vi "Write States.vi"(8 "error in (no error)":errorcluster, 10 "States":T1, 11 "MarkerTactic in":refnum<class "MarkerTactic.lvclass">) -> (0 "error out":errorcluster, 3 "MarkerTactic out":refnum<class "MarkerTactic.lvclass">)   [LabVIEW 2023, in "MarkerTactic.lvclass"]
uses:
  MarkerTactic.lvclass
  MarkerTacticStates.ctl
  MarkerTactic.lvclass/MarkerTactic.ctl
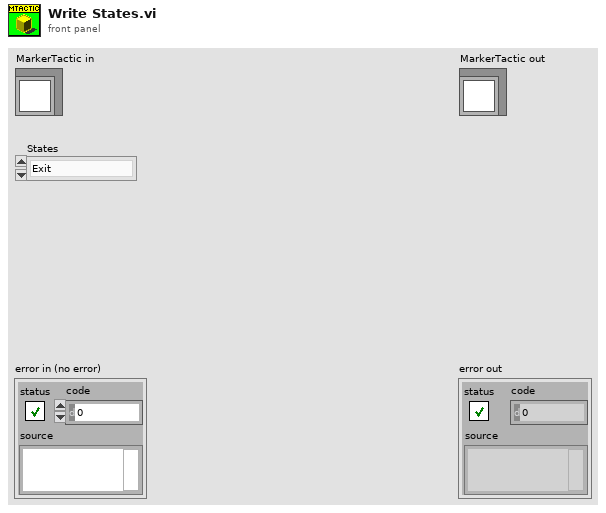
[diagram p1: front panel]
types:
  T1 = typedef "MarkerTacticStates.ctl" = enum16{"Exit", "BlockOurGoal", "FollowAttacker", "BlockEnemyPass"}
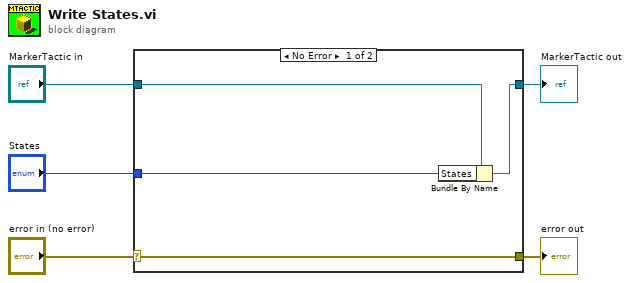
[diagram p0: block diagram]
diagram:
  n1 = case shown="No Error" "error in (no error)" {
    selector: "error in (no error)" -> [w9 w10]
    tunnel: [w9 w10] -> w4
    tunnel: [w7 w11] -> w2
    tunnel: "MarkerTactic in" -> [w8 w11]
    tunnel: "States" -> [w6 _]
    frame No Error {
      n2 = Bundle By Name(cluster=w8, "States"=w6) -> (w7:refnum<class "MarkerTactic.lvclass">)
    }
    frame Error {
    }
  }
  "error out" <- w4
  "MarkerTactic out" <- w2
